vi "Sub Bytes3.vi"(7 "Nb":i32=4, 8 "error in":errorcluster, 10 "State In":u16[][](array[numeric])=[[125, 216, 135, 144], [71, 71, 164, 177], [128, 52, 170, 55], [161, 141, 234, 198]]) -> (0 "error out":errorcluster, 2 "State Out":u16[][](array[numeric]))   [LabVIEW 2016, in "数据传输系统.lvlib"]
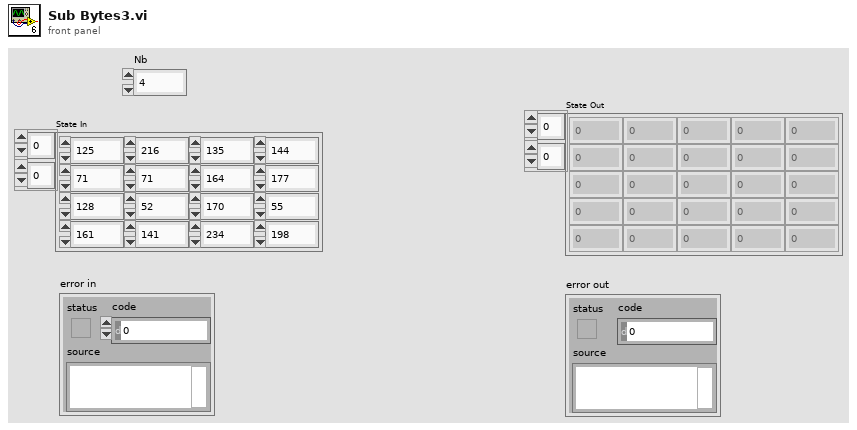
[diagram p1: front panel]
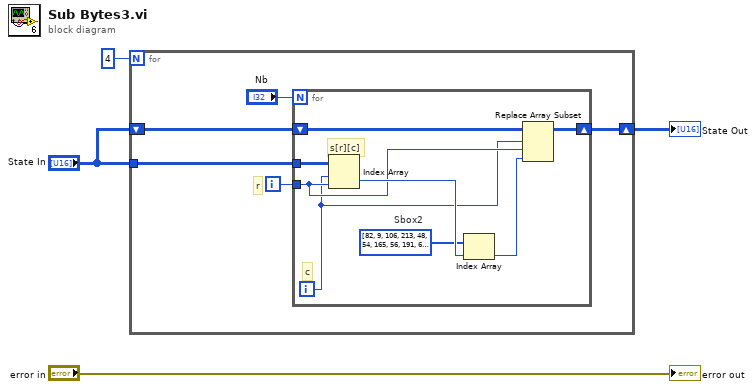
[diagram p0: block diagram]
diagram:
  n1 = for {
    N: 4 -> [_]
    tunnel: "State In" -> [w8]
    shift-right: [w5] -> w2
    shift-left: "State In" -> [w7]
    i -> [w9]
    # "r"
    n2 = for {
      N: "Nb" -> [_]
      tunnel: w8 -> [w17]
      tunnel: w9 -> [w14]
      shift-right: [w11] -> w5
      shift-left: w7 -> [w12]
      i -> [w13]
      w10 = i32[] [82, 9, 106, 213, 48, 54, 165, 56, 191, 64, 163, 158, 129, 243, 215, 251, 124, 227, 57, 130, 155, 47, 255, 135, 52, 142, 67, 68, 196, 222, 233, 203, 84, 123, 148, 50, 166, 194, 35, 61, 238, 76, 149, 11, 66, 250, 195, 78, 8, 46, 161, 102, 40, 217, 36, 178, 118, 91, 162, 73, 109, 139, 209, 37, 114, 248, 246, 100, 134, 104, 152, 22, 212, 164, 92, 204, 93, 101, 182, 146, 108, 112, 72, 80, 253, 237, 185, 218, 94, 21, 70, 87, 167, 141, 157, 132, 144, 216, 171, 0, 140, 188, 211, 10, 247, 228, 88, 5, 184, 179, 69, 6, 208, 44, 30, 143, 202, 63, 15, 2, 193, 175, 189, 3, 1, 19, 138, 107, 58, 145, 17, 65, 79, 103, 220, 234, 151, 242, 207, 206, 240, 180, 230, 115, 150, 172, 116, 34, 231, 173, 53, 133, 226, 249, 55, 232, 28, 117, 223, 110, 71, 241, 26, 113, 29, 41, 197, 137, 111, 183, 98, 14, 170, 24, 190, 27, 252, 86, 62, 75, 198, 210, 121, 32, 154, 219, 192, 254, 120, 205, 90, 244, 31, 221, 168, 51, 136, 7, 199, 49, 177, 18, 16, 89, 39, 128, 236, 95, 96, 81, 127, 169, 25, 181, 74, 13, 45, 229, 122, 159, 147, 201, 156, 239, 160, 224, 59, 77, 174, 42, 245, 176, 200, 235, 187, 60, 131, 83, 153, 97, 23, 43, 4, 126, 186, 119, 214, 38, 225, 105, 20, 99, 85, 33, 12, 125]  # Sbox2
      # "s[r][c]"
      # "c"
      n3 = Index Array(array=w17, index (row)=w13, index (col)=w14) -> (element=w16:u16)
      n4 = Index Array(array=w10, index=w16) -> (element=w15:i32)
      n5 = Replace Array Subset(array=w12, new element=w15, index (row)=w13, index (col)=w14) -> (w11:u16[][])
    }
  }
  "State Out" <- w2
  "error out" <- "error in"
